vi "Start.vi"(8 "Error In":errorcluster, 11 "reference in":refnum<class "NI9862.lvclass">) -> (0 "Error Out":errorcluster, 3 "reference out":refnum<class "NI9862.lvclass">)   [LabVIEW 2024, in "NI9862.lvclass"]
uses:
  NI9862.lvclass
  NI9862.lvclass/NI9862.ctl
  Source/Interfaces/IRunnable/IRunnable.lvclass
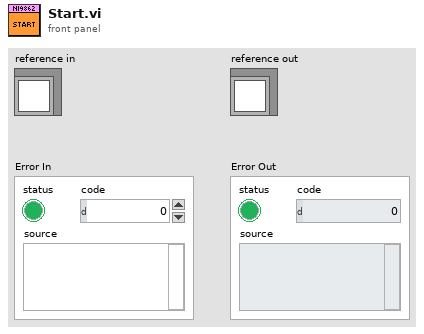
[diagram p1: front panel]
types:
  T1 = typedef "NI9862.lvclass/ObjectAttributes.ctl" = cluster{"IConfigure":refnum<class "IConfigure.lvclass">}
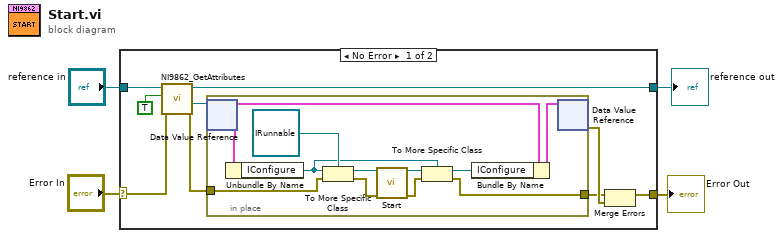
[diagram p0: block diagram]
diagram:
  n1 = case shown="No Error" "Error In" {
    selector: "Error In" -> [w12 w26]
    tunnel: [w9 w26] -> w3
    tunnel: [w10 w25] -> w1
    tunnel: "reference in" -> [w13 w25]
    frame No Error {
      n2 = call "NI9862_GetAttributes.vi"("Error In"=w12, "OnlyGetDvrReference(False)"=TRUE, "NI9862 in"=w13) -> ("Error Out"=w6:errorcluster, "DataRef"=w8:refnum<data-value>, "NI9862 out"=w10:refnum<class "NI9862.lvclass">)  [unwired: 5 in, 1 out]
      n3 = in-place {
        in-place-border: w6 -> [w15]
        in-place-border: [w14] -> w5
        n4 = in-place-dvr #1(w8) -> (w23:T1)  [unwired: 1 out]
        n5 = Unbundle By Name(w23) -> ("IConfigure"=w17:refnum<class "IConfigure.lvclass">)
        n6 = To More Specific Class(target class=refnum<class "IRunnable.lvclass"> refnum ("IRunnable.lvclass"), reference=w17, error in=w15) -> (specific class reference=w21:refnum<class "IRunnable.lvclass">, error out=w20:errorcluster)
        n7 = call-dynamic "Start.vi"("error in"=w20, "IRunnable in"=w21) -> ("error out"=w16:errorcluster, "IRunnable out"=w19:refnum<class "IRunnable.lvclass">)  [unwired: 8 in]
        n8 = To More Specific Class(target class=w17, reference=w19, error in=w16) -> (specific class reference=w18:refnum<class "IConfigure.lvclass">, error out=w14:errorcluster)
        n9 = Bundle By Name(cluster=w23, "IConfigure"=w18) -> (w24:T1)
        n10 = in-place-dvr #1(w24) -> (w11:errorcluster)  [unwired: 1 out]
      }
      n11 = Merge Errors(w5, w11) -> (w9:errorcluster)
    }
    frame Error {
    }
  }
  "Error Out" <- w3
  "reference out" <- w1
